vi "Delete Old Library from Project.vi"(8 "error in (no error)":errorcluster, 10 "folder to delete":string, 11 "path to project":path) -> (0 "error out":errorcluster)   [LabVIEW 2020]
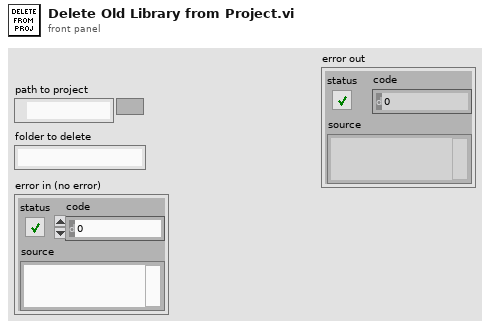
[diagram p1: front panel]
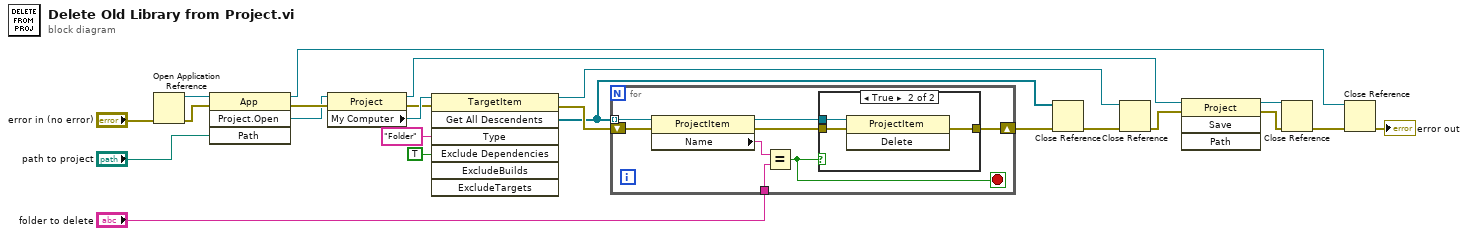
[diagram p0: block diagram]
diagram:
  n1 = Open Application Reference(8:"error in (no error)") -> (0:w17:errorcluster, 3:w16:refnum<vi>)  [unwired: 3 in]
  n2 = invoke class="App" method="Project.Open"(reference=w16, error in=w17, "Path"="path to project") -> (reference out=w7:refnum<vi>, error out=w20:errorcluster, "Project:Open"=w19:refnum<vi>)  [unwired: 1 in, 1 out]
  n3 = property class="Project"(reference=w19, error in=w20) -> (reference out=w6:refnum<vi>, error out=w21:errorcluster, "My Computer"=w22:refnum<vi>)
  n4 = invoke class="TargetItem" method="Get All Descendents"(reference=w22, error in=w21, "Type"="Folder", "Exclude Dependencies"=TRUE ("ExcludeDependencies")) -> (reference out=w10:refnum<vi>, error out=w14:errorcluster, "All Descendents"=w2:refnum<vi>[])  [unwired: 3 in, 4 out]
  n5 = for {
    tunnel: w2 -> [w31] mode=indexing
    shift-right: [w27] -> w12
    shift-left: w14 -> [w30]
    tunnel: "folder to delete" -> [w29]
    stop <- w24 stop-if-true
    n6 = property class="ProjectItem"(reference=w31, error in=w30) -> (reference out=w28:refnum<vi>, error out=w26:errorcluster, "Name"=w25:string)
    n7 = Equal?(x=w25, y=w29) -> (x = y?=w24:bool)
    n8 = case shown="True" w24 {
      tunnel: w28 -> [_ w35]
      tunnel: [w32 w34] -> w27
      tunnel: w26 -> [w32 w33]
      frame False {
      }
      frame True {
        n9 = invoke class="ProjectItem" method="Delete"(reference=w35, error in=w33) -> (error out=w34:errorcluster)  [unwired: 1 in, 2 out]
      }
    }
  }
  n10 = Close Reference(reference=w2, error in (no error)=w12) -> (error out=w11:errorcluster)
  n11 = Close Reference(reference=w10, error in (no error)=w11) -> (error out=w4:errorcluster)
  n12 = invoke class="Project" method="Save"(reference=w6, error in=w4) -> (reference out=w5:refnum<vi>, error out=w3:errorcluster)  [unwired: 2 in, 2 out]
  n13 = Close Reference(reference=w5, error in (no error)=w3) -> (error out=w9:errorcluster)
  n14 = Close Reference(reference=w7, error in (no error)=w9) -> (error out=→"error out":errorcluster)
